vi "setWavelength.vi"(8 "error in (no error)":errorcluster, 10 "wavelength":T2=4.0000000000000003e-07, 11 "MonoClientCommunicator in":refnum<class "MonoClientCommunicator.lvclass">) -> (0 "error out":errorcluster, 2 "ack":T1, 3 "MonoClientCommunicator out":refnum<class "MonoClientCommunicator.lvclass">)   [LabVIEW 2016, in "MonoClientCommunicator.lvclass"]
uses:
  MonoClientCommunicator.lvclass
  Typedefs/wavelength.ctl
  Typedefs/AckType.ctl
  Typedefs/MonoCommand.ctl
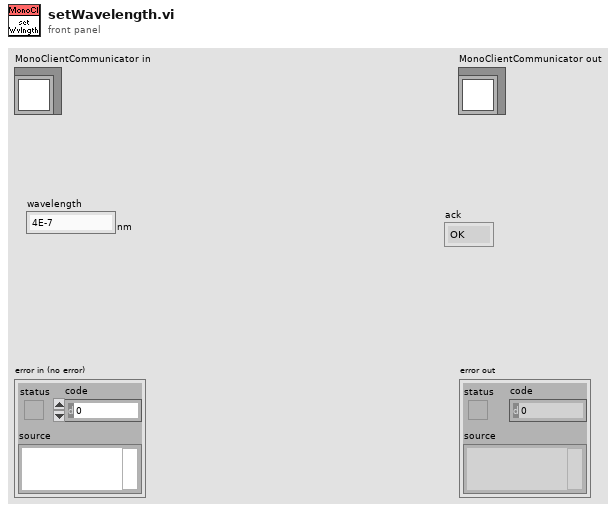
[diagram p1: front panel]
types:
  T1 = typedef "AckType.ctl" = enum16{"OK", "OutOfRange", "Unknown", "Busy", "Rejected"}
  T2 = typedef "wavelength.ctl" = dbl[unit]
  T3 = typedef "MonoCommand.ctl" = enum16{"getGrating", "getFrontEntranceSlitPosition", "getFrontExitSlitPosition", "getWavelength", "setWavelength", "setGrating", "setFrontEntranceSlitPosition", "setFrontExitSlitPosition", "calibrateWavelength", "getStatus", "Unknown", "reset"}
  T4 = typedef "publishers.ctl" = enum16{"Wavelength", "Grating", "FrontEntranceSlitPosition", "FrontExitSlitPosition", "SoftwareStatus", "MonochromatorId", "Ack"}
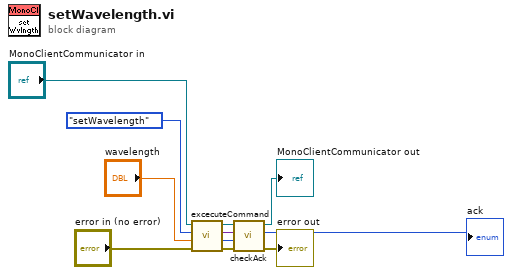
[diagram p0: block diagram]
diagram:
  n1 = call "excecuteCommand.vi"("error in (no error)"="error in (no error)", "input"="wavelength", "MonoCommand"=MonoCommand."setWavelength", "MonoClientCommunicator in"="MonoClientCommunicator in") -> ("error out"=w7:errorcluster, "parameter"=w10:T4, "value"=w9:variant, "MonoClientCommunicator out"=w8:refnum<class "MonoClientCommunicator.lvclass">)  [unwired: 4 in]
  n2 = call "checkAck.vi"("error in (no error)"=w7, "type"=w10, "value"=w9, "MonoClientCommunicator in"=w8) -> ("error out"=→"error out":errorcluster, "ack"=→"ack":T1, "MonoClientCommunicator out"=→"MonoClientCommunicator out":refnum<class "MonoClientCommunicator.lvclass">)  [unwired: 5 in]
